vi "Prabhakant_Find_Serial_Port.vi"(8 "error in (no error)":errorcluster) -> (0 "error out":errorcluster, 3 "Array":string[](array[string]))   [LabVIEW 2018]
doc: "This VI finds the VISA Resource Names of all COM ports on the host machine. It first finds the VISA Resource Names of all serial ports and then filters through these to find which of those are COM ports."
panel:
  out "Resource Names of All COM Devices Found":string[](array[string])
  out "Number of COM Resources Found":i32
  # "Find VISA COM Resource Names:\nThis VI finds the VISA Resource Names of all\nCOM ports on the host machine.  Just run the VI\nto find how many COM ports are found and to\nobtain an array of their VISA Resource Names."
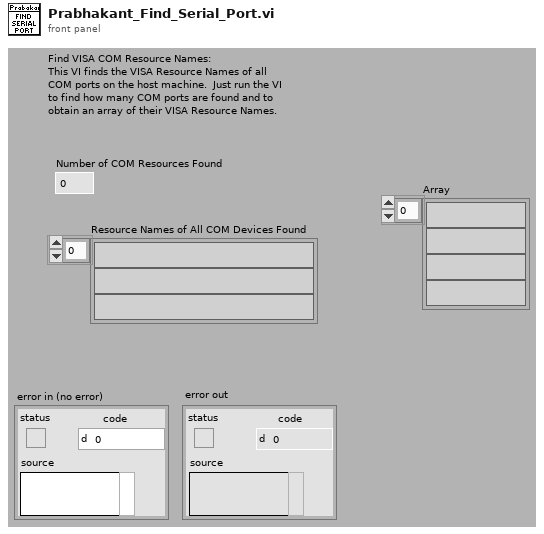
[diagram p1: front panel]
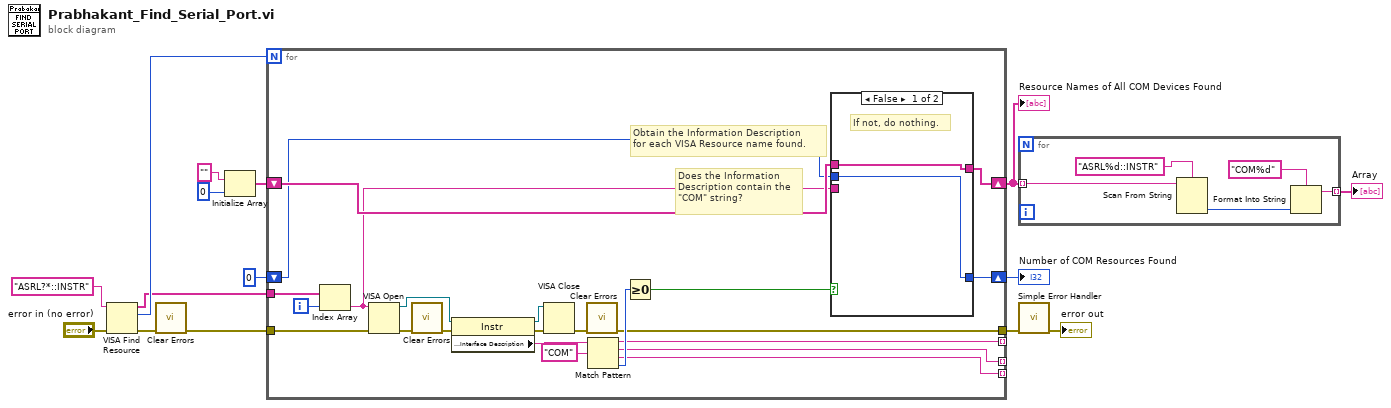
[diagram p0: block diagram]
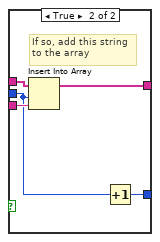
[diagram p2: hidden frame]
diagram:
  n1 = VISA Find Resource(8:"error in (no error)", 11:"ASRL?*::INSTR" ("expression (\"\")")) -> (0:w9:errorcluster, 2:w14:u32, 3:w13:string[])  [unwired: 1 in]
  n2 = call <vilib>:"Clear Errors.vi"("error in (no error)"=w9) -> ("error out"=w1:errorcluster)  [unwired: 5 in, 1 out]
  n3 = Initialize Array("", 0 ("dimension size")) -> (w10:string[])
  n4 = for {
    N: w14 -> [_]
    tunnel: w13 -> [w34]
    shift-right: [w26] -> w3
    shift-left: w10 -> [w29]
    tunnel: w1 -> [w25]
    tunnel: [w16] -> w8
    shift-right: [w22] -> w4
    shift-left: 0 -> [w23]
    tunnel: [w20] -> _ mode=indexing
    tunnel: [w19] -> _ mode=indexing
    tunnel: [w18] -> _ mode=indexing
    i -> [w30]
    # "Obtain the Information Description\nfor each VISA Resource name found."
    # "Does the Information \nDescription contain the\n\"COM\" string?"
    n5 = Index Array(array=w34, index=w30) -> (element=w27:string)
    n6 = VISA Open(error in (no error)=w25, VISA resource name=w27) -> (VISA resource name=w28:refnum<visa-resource-name>, error out=w36:errorcluster)  [unwired: 3 in]
    n7 = call <vilib>:"Clear Errors.vi"("error in (no error)"=w36) -> ("error out"=w17:errorcluster)  [unwired: 5 in, 1 out]
    n8 = property class="Instr"(reference=w28, error in=w17) -> (reference out=w37:refnum<visa-resource-name>, error out=w35:errorcluster, "Interface Information:Interface Description"=w21:string)
    n9 = VISA Close(VISA resource name=w37, error in (no error)=w35) -> (error out=w24:errorcluster)
    n10 = call <vilib>:"Clear Errors.vi"("error in (no error)"=w24) -> ("error out"=w16:errorcluster)  [unwired: 5 in, 1 out]
    n11 = Match Pattern(string=w21, regular expression="COM") -> (before substring=w20:string, match substring=w19:string, after substring=w18:string, offset past match=w32:i32)  [unwired: 1 in]
    n12 = Greater Or Equal To 0?(x=w32) -> (x >= 0?=w31:bool)
    n13 = case shown="False" w31 {
      tunnel: w23 -> [w38 w41]
      tunnel: [w39 w44] -> w26
      tunnel: w29 -> [w39 w43]
      tunnel: w27 -> [_ w42]
      tunnel: [w38 w40] -> w22
      frame False {
        # "If not, do nothing."
      }
      frame True {
        # "If so, add this string\nto the array"
        n14 = Insert Into Array(array=w43, index=w41, new element=w42) -> (w44:string[])
        n15 = Increment(x=w41) -> (x+1=w40:i32)
      }
    }
  }
  "Number of COM Resources Found" <- w4
  "Resource Names of All COM Devices Found" <- w3
  n16 = for {
    tunnel: w3 -> [w46] mode=indexing
    tunnel: [w45] -> w2 mode=indexing
    n17 = Scan From String(format string="ASRL%d::INSTR", input string=w46) -> (output 1=w47:i32)  [unwired: 3 in, 3 out]
    n18 = Format Into String(format string="COM%d" ("regular expression"), w47) -> (resulting string=w45:string)  [unwired: 2 in, 1 out]
  }
  "Array" <- w2
  n19 = call <vilib>:"Simple Error Handler.vi"("error in (no error)"=w8) -> ("error out"=→"error out":errorcluster)  [unwired: 4 in, 4 out]
